vi "Find script.vi"(8 "error in (no error)":errorcluster, 10 "Script name":string, 11 "Kasli":refnum<class "Kasli.lvclass">=refnum) -> (0 "error out":errorcluster, 2 "Found?":bool, 3 "Script path":path)   [LabVIEW 2020, in "CIRCUS_uServices.lvlib" / "Kasli Wrapper 2.0.lvlib" / "Kasli.lvclass"]
doc: "Vi for finding paths of scripts updated directly from the GUI. The entry is updated if the path is found. Otherwise the entry is deleted from the array. It looks for the scripts in th <ARTIQ_Codes>\\Scripts path and ignores Archive folders."
uses:
  Kasli.lvclass
  TALOS/TALOS_PPL.lvlibp
panel:
  out "path":path
  out "Indices":i32[](array[numeric])
  out "Paths":string[](array[string])
  # "For debug only"
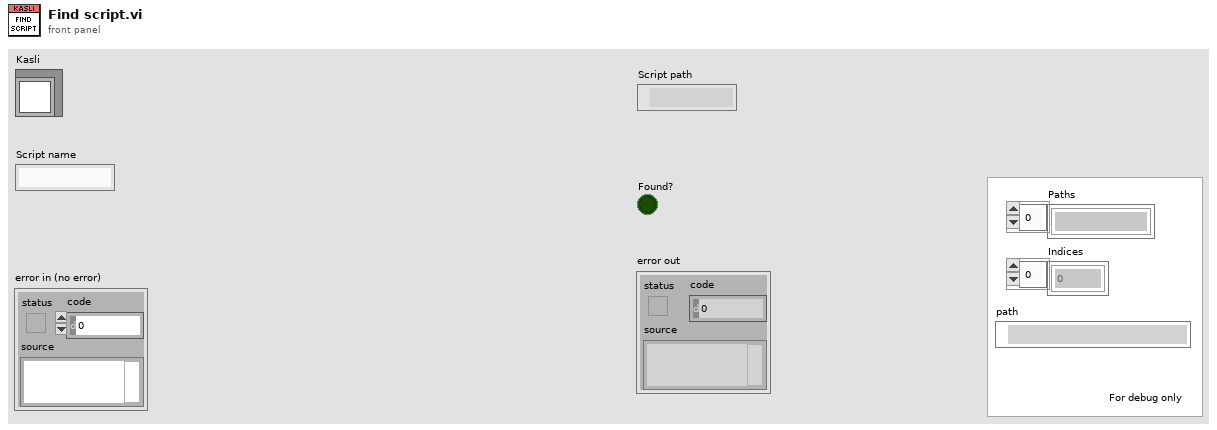
[diagram p1: front panel]
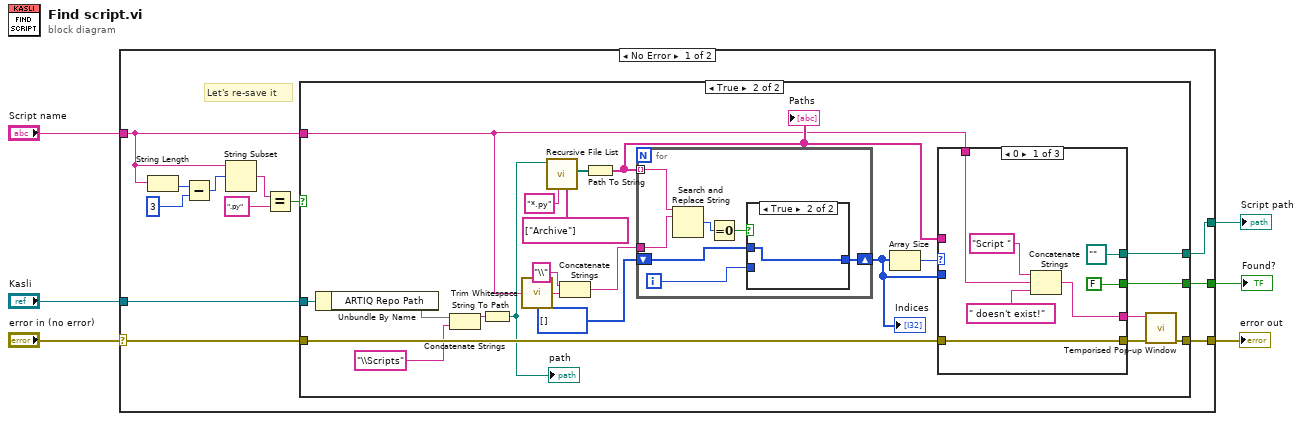
[diagram p0: block diagram]
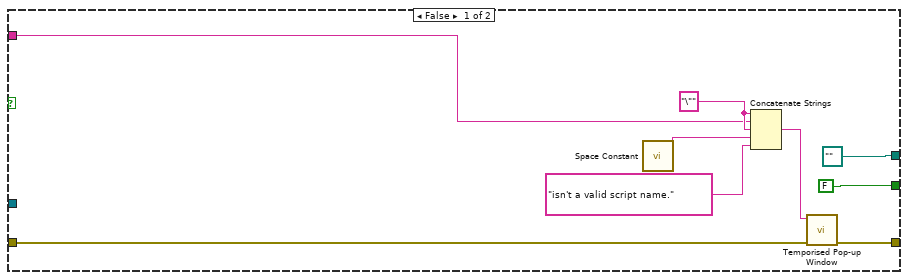
[diagram p2: hidden frame]
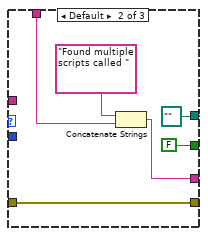
[diagram p3: hidden frame]
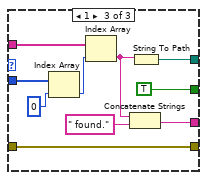
[diagram p4: hidden frame]
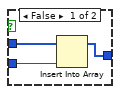
[diagram p5: hidden frame]
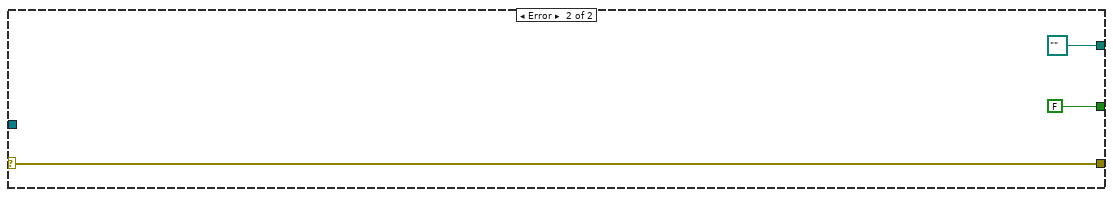
[diagram p6: hidden frame]
diagram:
  n1 = case shown="No Error" "error in (no error)" {
    selector: "error in (no error)" -> [w18 w86]
    tunnel: [w16 FALSE] -> w4
    tunnel: [w17 w86] -> w5
    tunnel: "Script name" -> [w8 _]
    tunnel: [w15 path ""] -> w2
    tunnel: "Kasli" -> [w14 _]
    frame No Error {
      # "Let's re-save it"
      n2 = String Length(string=w8) -> (length=w13:i32)
      n3 = Subtract(x=w13, y=3) -> (x-y=w11:i32)
      n4 = String Subset(string=w8, offset (0)=w11) -> (substring=w10:string)  [unwired: 1 in]
      n5 = Equal?(x=w10, y=".py") -> (x = y?=w7:bool)
      n6 = case shown="True" w7 {
        tunnel: w18 -> [w23 w49]
        tunnel: [path "" w39] -> w15
        tunnel: [FALSE w38] -> w16
        tunnel: [w24 w29] -> w17
        tunnel: w8 -> [w19 w33]
        tunnel: w14 -> [_ w32]
        frame False {
          w20 = "\"" ("string")
          n7 = call <vilib>:"Space Constant.vi"() -> ("String"=w22:string)
          n8 = Concatenate Strings(w20, w19, w20, w22, "isn't a valid script name." ("string")) -> (w27:string)
          n9 = call "Temporised Pop-up Window.vi"("error in (no error)"=w23, "Text"=w27) -> ("error out"=w24:errorcluster)  [unwired: 9 in]
        }
        frame True {
          n10 = Unbundle By Name(w32) -> ("ARTIQ Repo Path"=w31)
          n11 = Concatenate Strings(w31, "\\Scripts" ("string")) -> (w36:string)
          n12 = String To Path(string=w36) -> (path=w42:path)
          "path" <- w42
          n13 = call <vilib>:"Trim Whitespace.vi"("string"=w33) -> ("trimmed string"=w37:string)  [unwired: 1 in]
          n14 = call <vilib>:"Recursive File List.vi"("Folders to Exclude"=string[] ["Archive"], "pattern"="*.py", "Folder Path"=w42) -> ("All Files in Dir"=w47:path[])  [unwired: 4 in, 4 out]
          n15 = Concatenate Strings("\\" ("string"), w37) -> (w40:string)
          n16 = Path To String(path=w47) -> (string=w44:string[])
          "Paths" <- w44
          n17 = for {
            tunnel: w44 -> [w76] mode=indexing
            tunnel: w40 -> [w75]
            shift-right: [w77] -> w43
            shift-left: i32[] [] -> [w78]
            i -> [w79]
            n18 = Search and Replace String(input string=w76, search string=w75) -> (number of replacements=w73:i32)  [unwired: 6 in, 3 out]
            n19 = Equal To 0?(x=w73) -> (x = 0?=w74:bool)
            n20 = case shown="True" w74 {
              tunnel: w79 -> [w80 _]
              tunnel: w78 -> [w82 w83]
              tunnel: [w81 w83] -> w77
              frame False {
                n21 = Insert Into Array(array=w82, new element=w80) -> (w81:i32[])  [unwired: 1 in]
              }
              frame True {
              }
            }
          }
          "Indices" <- w43
          n22 = Array Size(array=w43) -> (size(s)=w45:i32)
          n23 = case shown="0" w45 {
            tunnel: w44 -> [_ _ w69]
            tunnel: w43 -> [_ _ w72]
            tunnel: [path "" path "" w68] -> w39
            tunnel: [FALSE FALSE TRUE] -> w38
            tunnel: [w50 w58 w63] -> w30
            tunnel: w49 -> [w50 w58 w63]
            tunnel: w33 -> [w52 w59 _]
            tunnel: [w51 w57 w64] -> w28
            frame 0 {
              n24 = Concatenate Strings("Script " ("string"), w52, " doesn't exist!") -> (w51:string)
            }
            frame Default {
              n25 = Concatenate Strings("Found multiple scripts called " ("string"), w59) -> (w57:string)
            }
            frame 1 {
              n26 = Index Array(array=w72, index=0) -> (element=w70:i32)
              n27 = Index Array(array=w69, index=w70) -> (element=w67:string)
              n28 = Concatenate Strings(w67, " found." ("string")) -> (w64:string)
              n29 = String To Path(string=w67) -> (path=w68:path)
            }
          }
          n30 = call "Temporised Pop-up Window.vi"("error in (no error)"=w30, "Text"=w28) -> ("error out"=w29:errorcluster)  [unwired: 9 in]
        }
      }
    }
    frame Error {
    }
  }
  "error out" <- w5
  "Found?" <- w4
  "Script path" <- w2
